vi "CommsTestLoop.vi"() -> (2 "Pressure(hPa)":dbl format="%.1f")   [LabVIEW 2017]
panel:
  out "Case":string
  out "Array - String":string[](array[string])
  out "loops":i32
  in  "timeout ms":i32=2000
  in  "remote port or service name":u16=2000
  in  "address":string="192.168.126.101"
  in  "data in":string="*SRHb\n"
  out "data out":string
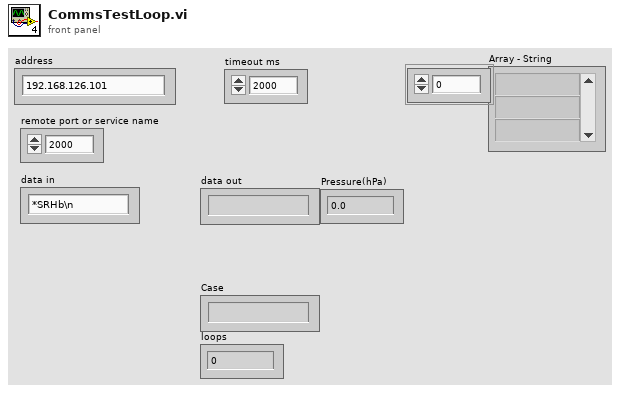
[diagram p1: front panel]
types:
  T1 = enum16{"Standard", "Buffered", "CRLF", "Immediate"}
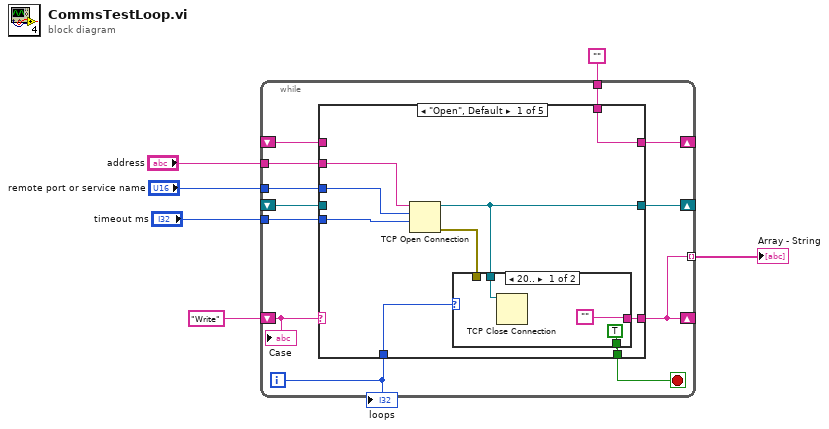
[diagram p0: block diagram]
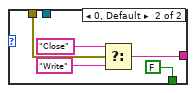
[diagram p2: hidden frame]
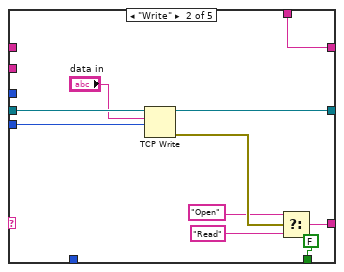
[diagram p3: hidden frame]
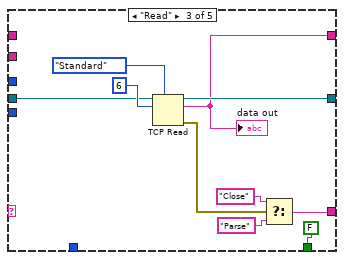
[diagram p4: hidden frame]
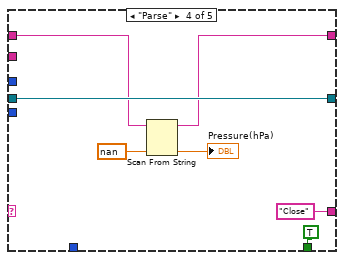
[diagram p5: hidden frame]
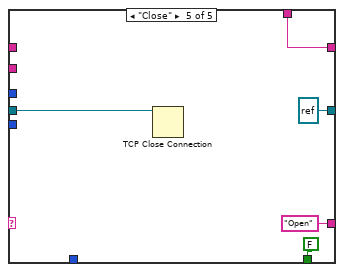
[diagram p6: hidden frame]
diagram:
  n1 = while {
    shift-right: [w7] -> _
    shift-left: "Write" -> [w18]
    tunnel: "timeout ms" -> [w17]
    tunnel: "address" -> [w16]
    shift-right: [w15] -> _
    shift-left: _ -> [w14]
    tunnel: "remote port or service name" -> [w13]
    shift-right: [w12] -> _
    shift-left: _ -> [w10]
    tunnel: "" -> [w11]
    tunnel: [w7] -> w1 mode=indexing
    i -> [w8]
    stop <- w9 stop-if-true
    n2 = case shown="\"Open\", Default" w18 {
      tunnel: [w24 w41 w49 "Close" "Open"] -> w7
      tunnel: w17 -> [w27 w38 _ _ _]
      tunnel: w16 -> [w26 _ _ _ _]
      tunnel: [w19 w44 w52 w62 refnum<k5> refnum ("connection ID")] -> w15
      tunnel: w14 -> [_ w45 w53 w62 w67]
      tunnel: w13 -> [w25 _ _ _ _]
      tunnel: [w22 w37 w51 w56 w64] -> w12
      tunnel: w11 -> [w22 w37 _ _ w64]
      tunnel: w10 -> [_ _ _ w59 _]
      tunnel: [w21 FALSE FALSE TRUE FALSE] -> w9
      tunnel: w8 -> [w20 _ _ _ _]
      frame "Open", Default {
        n3 = TCP Open Connection(address=w26, remote port or service name=w25, timeout ms (60000)=w27) -> (connection ID=w19:refnum<k5>, error out=w23:errorcluster)  [unwired: 2 in]
        n4 = case shown="20.." w20 {
          tunnel: ["" w35] -> w24
          tunnel: w23 -> [_ w34]
          tunnel: [TRUE FALSE] -> w21
          tunnel: w19 -> [w30 _]
          frame 20.. {
            n5 = TCP Close Connection(connection ID=w30) -> ()  [unwired: 2 in, 2 out]
          }
          frame 0, Default {
            n6 = Select(t="Close", s=w34, f="Write") -> (s? t:f=w35:string)
          }
        }
      }
      frame "Write" {
        n7 = TCP Write(connection ID=w45, data in="data in", 9:w38) -> (connection ID out=w44:refnum<k5>, error out=w42:errorcluster)  [unwired: 1 in, 1 out]
        n8 = Select(t="Open", s=w42, f="Read") -> (s? t:f=w41:string)
      }
      frame "Read" {
        n9 = TCP Read(connection ID=w53, bytes to read=6, 7:T1."Standard" ("mode (standard)")) -> (connection ID out=w52:refnum<k5>, data out=w51:string, error out=w48:errorcluster)  [unwired: 2 in]
        "data out" <- w51
        n10 = Select(t="Close", s=w48, f="Parse") -> (s? t:f=w49:string)
      }
      frame "Parse" {
        n11 = Scan From String(input string=w59, default 1=nan ("default value 1")) -> (remaining string=w56:string, output 1=→"Pressure(hPa)":dbl)  [unwired: 3 in, 2 out]
      }
      frame "Close" {
        n12 = TCP Close Connection(connection ID=w67) -> ()  [unwired: 2 in, 2 out]
      }
    }
    "loops" <- w8
    "Case" <- w18
  }
  "Array - String" <- w1
